vi "test harness_FXP_K_times_X_single_axis.vi"(8 "error in (no error)":errorcluster, 11 "TestCase in":refnum<class "FXP_observer_TestCase.lvclass">) -> (0 "error out":errorcluster, 3 "TestCase out":refnum<class "FXP_observer_TestCase.lvclass">)   [LabVIEW 2017, in "FXP_observer_TestCase.lvclass"]
uses:
  FXP_observer_TestCase.lvclass
  <vilib>/rvi/DesktopExecutionNode/Execution/niFpgaDEN_Execute.vi
  <vilib>/rvi/DesktopExecutionNode/DesktopExecutionNode.xnode
  <vilib>/addons/_JKI Toolkits/VI Tester/TestCase.llb/TestCase.lvclass
  C:/Program Files (x86)/National Instruments/LabVIEW 2017/vi.lib/addons/_JKI Toolkits/VI Tester/TestCase.llb/TestCase.lvclass
panel:
  out "xvec":fxp<+/-,32,6>[](array[numeric])
  in  "yd_est_x":fxp<+/-,32,5>
  in  "Nbar":fxp<+/-,32,5>
  in  "ref":fxp<+/-,32,5>
  out "K*x":dbl
  in  "xerr":fxp<+/-,32,5>[](array[numeric])=[1.0, 2.0, 5.0, 2.0, 0.0, 0.0, 0.0, 0.0, 0.0, 0.0, 0.0, 0.0, 0.0, 0.0, 0.0, 0.0, 0.0, 0.0, 0.0, 0.0, 0.0, 0.0, 0.0, 0.0, 0.0, 0.0, 0.0, 0.0, 0.0, 0.0, 0.0, 0.0, 0.0, 0.0, 0.0, 0.0, 0.0, 0.0, 0.0, 0.0, 0.0, 0.0, 0.0, 0.0, 0.0, 0.0, 0.0, 0.0]
  in  "NS +1":u8=5
  out "K*x (expected)":dbl
  in  "K_lqr":fxp<+/-,32,5>[](array[numeric])=[10.0, 0.5, 0.20000000298023224, 0.20000000298023224, 0.29999999701976776, 2.0, 0.0, 0.0, 0.0, 0.0, 0.0, 0.0, 0.0, 0.0, 0.0, 0.0, 0.0, 0.0, 0.0, 0.0, 0.0, 0.0, 0.0, 0.0, 0.0, 0.0, 0.0, 0.0, 0.0, 0.0, 0.0, 0.0, 0.0, 0.0, 0.0, 0.0, 0.0, 0.0, 0.0, 0.0, 0.0, 0.0, 0.0, 0.0, 0.0, 0.0, 0.0, 0.0, 0.0, 0.0]
  in  "x":fxp<+/-,32,5>[](array[numeric])=[1.0, 2.0, 3.0, 2.0, 6.0, 8.0, 0.0, 0.0, 0.0, 0.0, 0.0, 0.0, 0.0, 0.0, 0.0, 0.0, 0.0, 0.0, 0.0, 0.0, 0.0, 0.0, 0.0, 0.0, 0.0, 0.0, 0.0, 0.0, 0.0, 0.0, 0.0, 0.0, 0.0, 0.0, 0.0, 0.0, 0.0, 0.0, 0.0, 0.0, 0.0, 0.0, 0.0, 0.0, 0.0, 0.0, 0.0, 0.0, 0.0, 0.0]
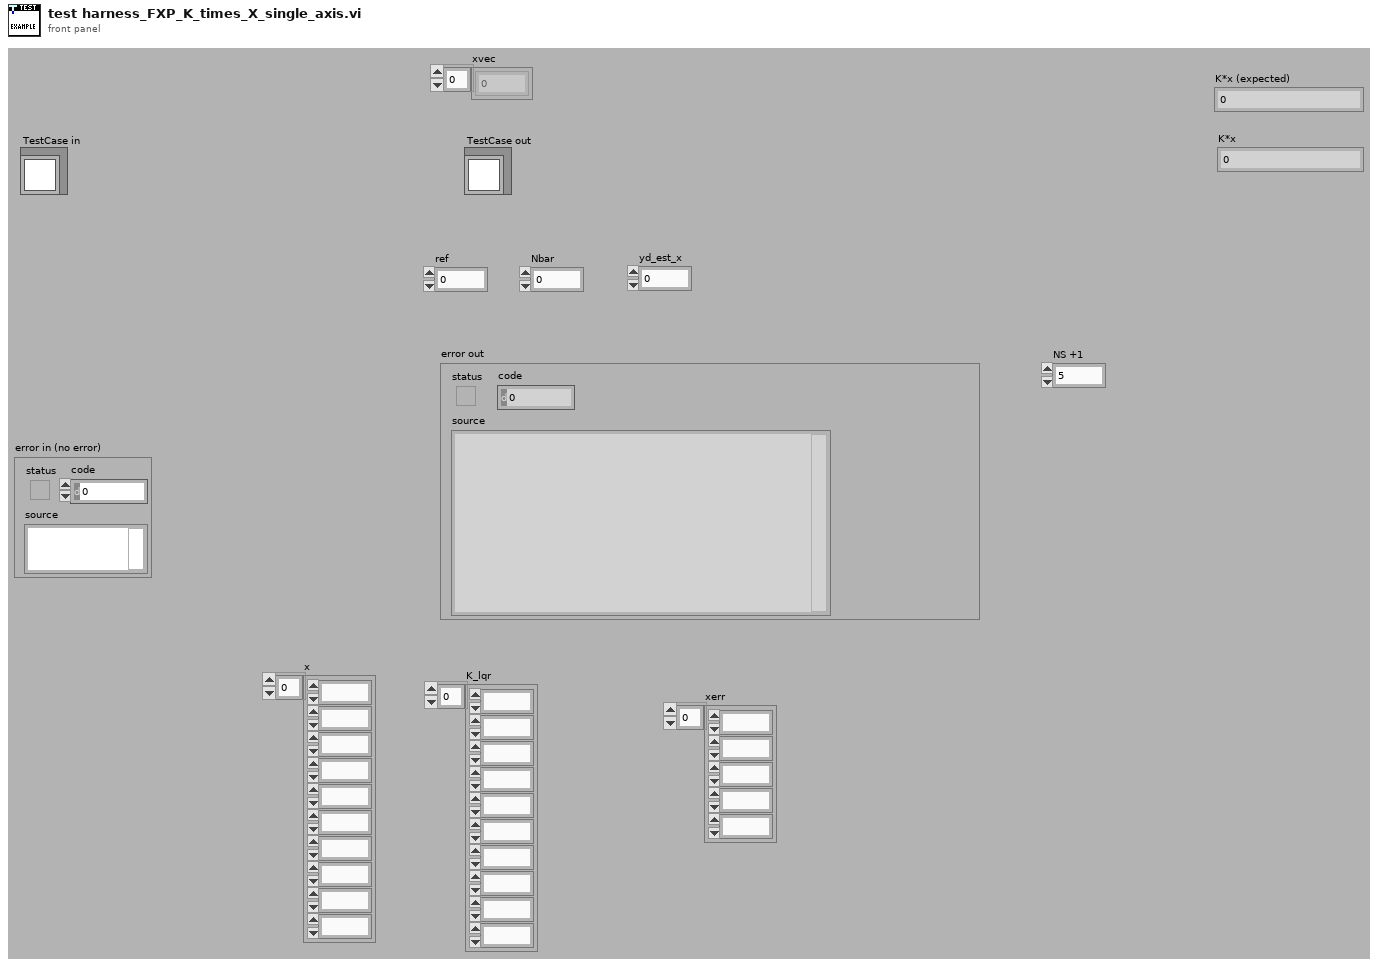
[diagram p1: front panel]
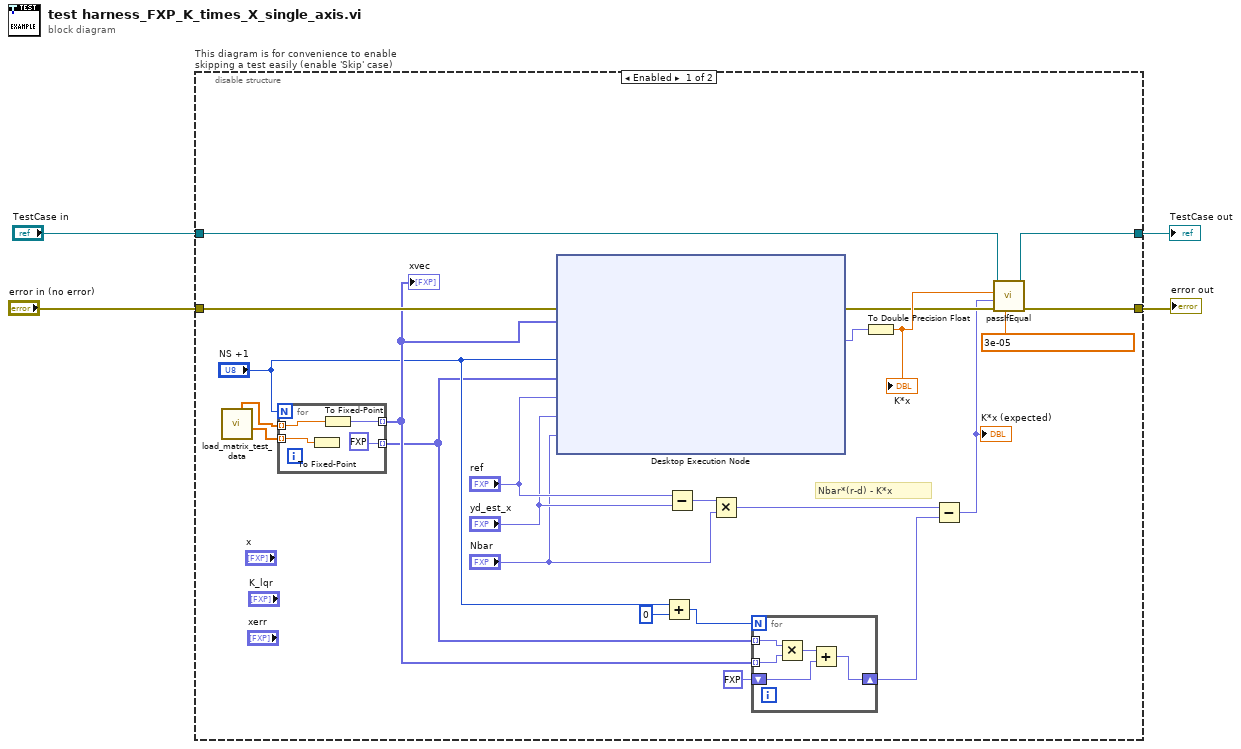
[diagram p0: block diagram]
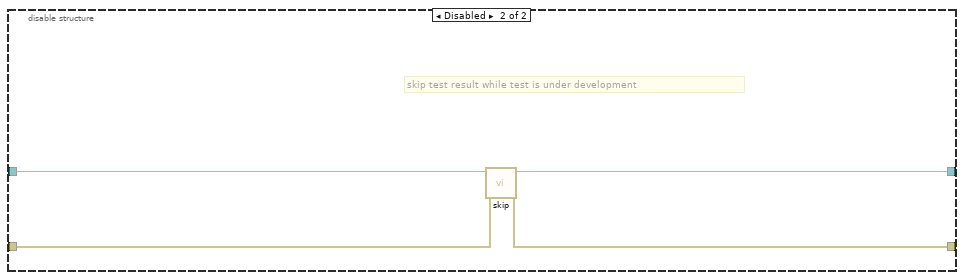
[diagram p2: hidden frame]
diagram:
  n1 = disable-structure "This diagram is for convenience to enable skipping a test easily (enable 'Skip' case)" shown="Enabled" {
    disable-tunnel: "TestCase in" -> [w27 w40]
    disable-tunnel: [w26 w38] -> w1
    disable-tunnel: [w25 w39] -> w3
    disable-tunnel: "error in (no error)" -> [w22 w37]
    frame Enabled {
      # "Nbar*(r-d) - K*x"
      n2 = call "load_matrix_test_data.vi"() -> ("Kz"=w20:dbl[], "X_test"=w16:dbl[])  [unwired: 4 in, 6 out]
      n3 = for {
        N: "NS +1" -> [_]
        tunnel: w20 -> [w36] mode=indexing
        tunnel: [fxp<+/-,32,6> 0.0 ("fixed-point")] -> w13 mode=indexing
        tunnel: w16 -> [w35] mode=indexing
        tunnel: [w34] -> w15 mode=indexing
        n4 = To Fixed-Point(number=w36) -> ()  [unwired: 1 in, 1 out]
        n5 = To Fixed-Point(number=w35) -> (fixed-point=w34:fxp<+/-,32,6>)  [unwired: 1 in]
      }
      "xvec" <- w15
      n6 = xnode "Desktop Execution Node"("Error In"=w22, "x_vec"=w15, "NS + 1"="NS +1", "K_lqr"=w13, "ref"="ref", "yd_est_x"="yd_est_x", "Nbar"="Nbar") -> ("Error Out"=w23:errorcluster, "del u_x"=w12:fxp<+/-,64,15>)
      n7 = Add(x="NS +1", y=i8 0) -> (x+y=w18:u8)
      n8 = Subtract(x="ref", y="yd_est_x") -> (x-y=w10:fxp<+/-,33,6>)
      n9 = Multiply(x=w10, y="Nbar") -> (x*y=w9:fxp<+/-,64,10>)
      n10 = for {
        N: w18 -> [_]
        tunnel: w13 -> [w31] mode=indexing
        tunnel: w15 -> [w30] mode=indexing
        shift-right: [w29] -> w8
        shift-left: fxp<+/-,32,5> 0.0 -> [w28]
        n11 = Multiply(x=w31, y=w30) -> (x*y=w32:fxp<+/-,64,12>)
        n12 = Add(x=w32, y=w28) -> (x+y=w29:fxp<+/-,64,10>)
      }
      n13 = To Double Precision Float(number=w12) -> (double precision float=w24:dbl)
      "K*x" <- w24
      n14 = Subtract(x=w9, y=w8) -> (x-y=w7:fxp<+/-,64,11>)
      "K*x (expected)" <- w7
      n15 = call-dynamic "passIfEqual.vi"("delta (optional)"=3e-05 ("del u_x"), "error in (no error)"=w23, "y"=w7, "x"=w24, "TestCase in"=w27) -> ("error out"=w25:errorcluster, "TestCase out"=w26:refnum<class "FXP_observer_TestCase.lvclass">)  [unwired: 5 in]
    }
    frame Disabled {
      # "skip test result while test is under development"
      n16 = call <vilib>:"skip.vi"("error in (no error)"=w37, "TestCase in"=w40) -> ("error out"=w39:errorcluster, "TestCase out"=w38:refnum<class "FXP_observer_TestCase.lvclass">)  [unwired: 8 in]
    }
  }
  "error out" <- w3
  "TestCase out" <- w1
